vi "Cylinder Kinematics Modification.vi"(1 "Radius":dbl, 2 "Max Velocity":dbl[](array[numeric])) -> (0 "Max Velocity Modified":dbl[](array[numeric]))   [LabVIEW 2014, in "Guidance Library.lvlib" / "Joystick Guidance.lvclass"]
uses:
  Joystick Guidance.lvclass
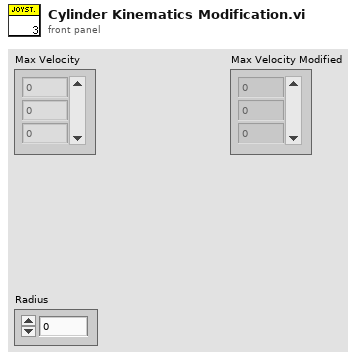
[diagram p1: front panel]
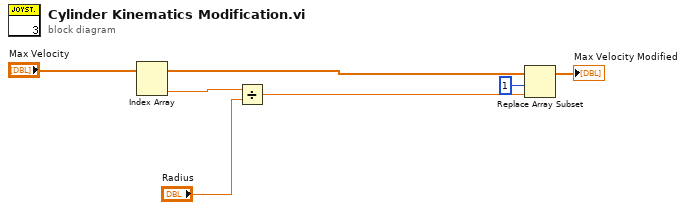
[diagram p0: block diagram]
diagram:
  n1 = Index Array(array="Max Velocity") -> (element #2=w5:dbl)  [unwired: 2 in, 1 out]
  n2 = Divide(x=w5, y="Radius") -> (x/y=w4:dbl)
  n3 = Replace Array Subset(array="Max Velocity", new element=w4, index=1) -> (→"Max Velocity Modified":dbl[])
